vi "set channel.vi"(8 "error in":errorcluster, 10 "channel":refnum<class "TBM channel.lvclass">, 11 "sample module configuration in":refnum<class "sample module configuration.lvclass">) -> (0 "error out":errorcluster, 3 "sample module configuration out":refnum<class "sample module configuration.lvclass">)   [LabVIEW 2013, in "sample module configuration.lvclass"]
doc: "This function is responsible for replacing a channel, by name in the configuration class."
uses:
  sample module configuration.lvclass
  channel/TBM channel.lvclass
  <vilib>/NI/Tag Bus/tag/tag descriptor.lvclass/tag descriptor.ctl
  sample module configuration.lvclass/sample module configuration.ctl
  <vilib>/NI/Tag Bus/tag/tag descriptor.lvclass
  root configuration/TBM configuration.lvclass
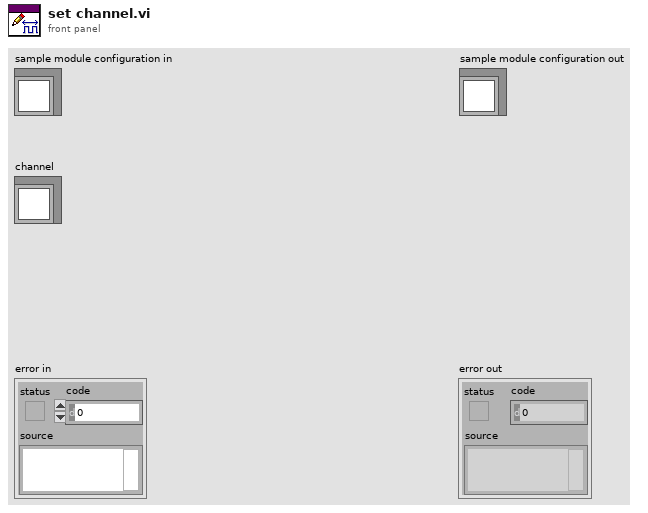
[diagram p1: front panel]
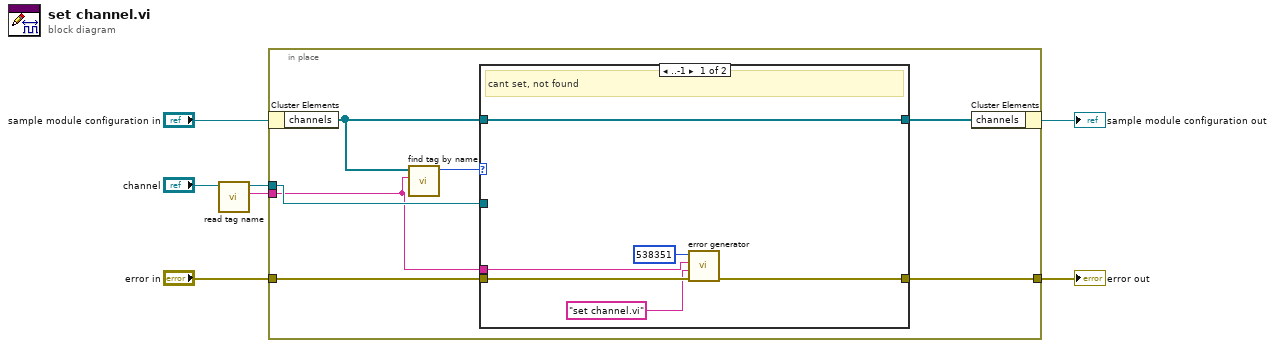
[diagram p0: block diagram]
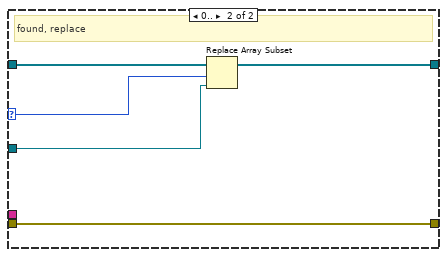
[diagram p2: hidden frame]
diagram:
  n1 = call <vilib>:"read tag name.vi"("system tag in"="channel") -> ("name"=w1:string, "system tag out"=w2:refnum<class "TBM channel.lvclass">)  [unwired: 8 in, 1 out]
  n2 = in-place {
    in-place-border: [w12] -> w5
    in-place-border: "error in" -> [w10]
    in-place-border: w2 -> [w9]
    in-place-border: w1 -> [w8]
    n3 = in-place-cluster #1("sample module configuration in") -> ("channels"=w13:refnum<class "TBM channel.lvclass">[])
    n4 = call <vilib>:"find tag by name.vi"("name"=w8, "tags in"=w13) -> ("index"=w14:i32)  [unwired: 9 in]
    n5 = case shown="..-1" w14 {
      selector: w14 -> [_ w21]
      tunnel: w13 -> [w18 w24]
      tunnel: [w19 w25] -> w12
      tunnel: [w18 w23] -> w11
      tunnel: w10 -> [w17 w25]
      tunnel: w9 -> [_ w22]
      tunnel: w8 -> [w16 _]
      frame ..-1 {
        # "cant set, not found"
        n6 = call "error generator.vi"("error in"=w17, "source"="set channel.vi", "append error message"=w16, "error code (0)"=538351) -> ("error out"=w19:errorcluster)  [unwired: 7 in]
      }
      frame 0.. {
        # "found, replace"
        n7 = Replace Array Subset(array=w24, new element=w22, index=w21) -> (w23:refnum<class "TBM channel.lvclass">[])
      }
    }
    n8 = in-place-cluster #1("channels"=w11) -> (→"sample module configuration out":refnum<class "sample module configuration.lvclass">)
  }
  "error out" <- w5
